vi "Poll Server.vi"() -> ()   [LabVIEW 2014]
uses:
  <vilib>/addons/zeromq/socket_type.ctl
  <userlib>/_OpenG.lib/numeric/numeric.llb/Random Number Within Range - DBL__ogtk.vi
  <vilib>/addons/zeromq/zmq_context.lvclass
  <vilib>/addons/zeromq/zeromq.lvlib
  <vilib>/addons/zeromq/zmq_socket.lvclass
panel:
  in  "stop":bool
  out "concatenated string":string
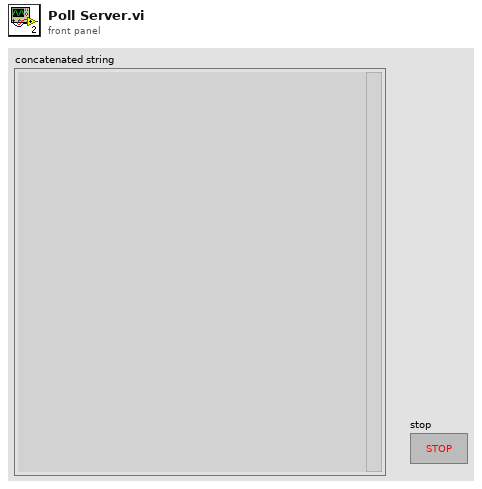
[diagram p1: front panel]
types:
  T1 = typedef "zeromq.lvlib/socket_type.ctl" = enum8{"ZMQ_PAIR", "ZMQ_PUB", "ZMQ_SUB", "ZMQ_REQ", "ZMQ_REP", "ZMQ_DEALER", "ZMQ_ROUTER", "ZMQ_PULL", "ZMQ_PUSH", "ZMQ_XPUB", "ZMQ_XSUB"}
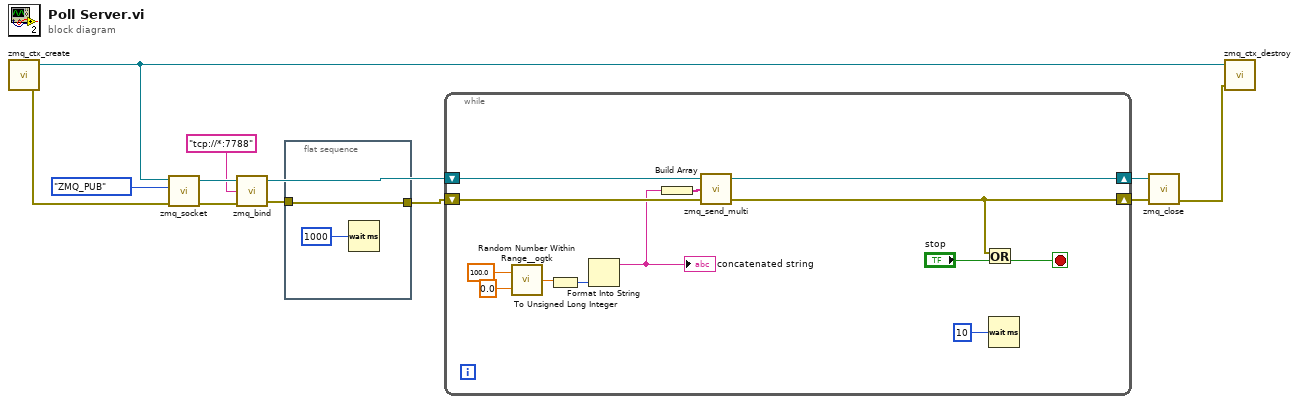
[diagram p0: block diagram]
diagram:
  n1 = call <vilib>:"zmq_ctx_create.vi"() -> ("error out"=w11:errorcluster, "context out"=w10:refnum<class "zmq_context.lvclass">)  [unwired: 4 in]
  n2 = call <vilib>:"zmq_socket.vi"("error in"=w11, "socket type"=socket_type."ZMQ_PUB", "context in"=w10) -> ("error out"=w8:errorcluster, "socket out"=w9:refnum<class "zmq_socket.lvclass">)  [unwired: 2 in, 1 out]
  n3 = call <vilib>:"zmq_bind.vi"("error in"=w8, "endpoint"="tcp://*:7788", "socket in"=w9) -> ("error out"=w1:errorcluster, "socket out"=w5:refnum<class "zmq_socket.lvclass">)  [unwired: 1 in]
  n4 = flat-sequence {
    tunnel: [w13] -> w2
    tunnel: w1 -> [w13]
    frame #0 {
      n5 = Wait (ms)(milliseconds to wait=u32 1000) -> ()  [unwired: 1 out]
    }
  }
  n6 = while {
    shift-right: [w26] -> w4
    shift-left: w5 -> [w27]
    shift-right: [w16] -> w3
    shift-left: w2 -> [w25]
    stop <- w17 stop-if-true
    n7 = call-poly <userlib>:"Random Number Within Range__ogtk.vi"("High"=100.0, "Low"=0.0) -> ("Random Number"=w22:dbl)  [unwired: 3 in]
    n8 = To Unsigned Long Integer(number=w22) -> (unsigned 32bit integer=w21:u32)
    n9 = Format Into String(w21) -> (resulting string=w20:string)  [unwired: 3 in, 1 out]
    "concatenated string" <- w20
    n10 = Build Array(w20) -> (w15:string[])
    n11 = call <vilib>:"zmq_send_multi.vi"("error in"=w25, "parts"=w15, "socket in"=w27) -> ("error out"=w16:errorcluster, "socket out"=w26:refnum<class "zmq_socket.lvclass">)  [unwired: 1 in]
    n12 = Or(x=w16, y="stop") -> (x .or. y?=w17:bool)
    n13 = Wait (ms)(milliseconds to wait=u32 10) -> ()  [unwired: 1 out]
  }
  n14 = call <vilib>:"zmq_close.vi"("error in"=w3, "socket"=w4) -> ("error out"=w6:errorcluster)  [unwired: 3 in]
  n15 = call <vilib>:"zmq_ctx_destroy.vi"("error in"=w6, "context in"=w10) -> ()  [unwired: 3 in, 1 out]
